vi "Release.vi"(8 "error in":errorcluster, 11 "Loop Data":T1={"VI Refnum"=refnum, "Timeout"=-1, "Code Data"=[], "Buffer Data"={"Connection ID"=refnum}, "Timer"=4294967295, "Image"=refnum}) -> (0 "error out":errorcluster)   [LabVIEW 2016]
uses:
  Data Def/Loop Data.ctl
  Com/Matrix220/Data Def/Com_Matrix220_Buffer Data.ctl
  <vilib>/vision/Image Controls.llb/IMAQ Image.ctl
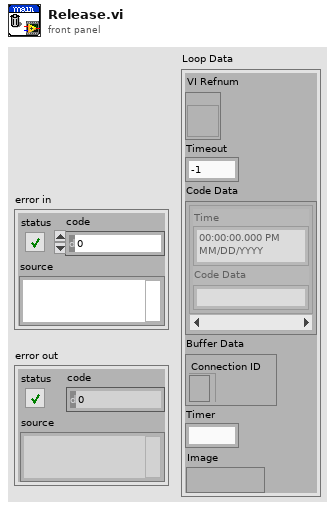
[diagram p1: front panel]
types:
  T1 = typedef "Loop Data.ctl" = cluster{"VI Refnum":refnum<vi>, "Timeout":i32, "Code Data":cluster{"Time":timestamp, "Code Data":string}[], "Buffer Data":T2, "Timer":u32, "Image":T3}
  T2 = typedef "Com_Matrix220_Buffer Data.ctl" = cluster{"Connection ID":refnum<k5>}
  T3 = typedef "IMAQ Image.ctl" = refnum<image>
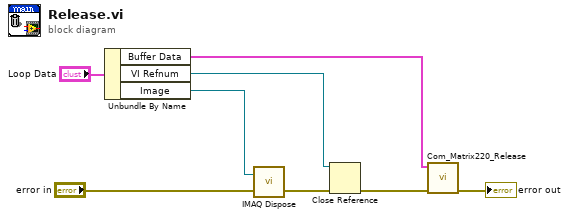
[diagram p0: block diagram]
diagram:
  n1 = Unbundle By Name("Loop Data") -> ("Buffer Data"=w5:T2, "VI Refnum"=w7:refnum<vi>, "Image"=w2:T3)
  n2 = call "IMAQ Dispose"("Image"=w2, "error in (no error)"="error in") -> ("error out"=w1:errorcluster)  [unwired: 4 in]
  n3 = Close Reference(reference=w7, error in (no error)=w1) -> (error out=w6:errorcluster)
  n4 = call "Com_Matrix220_Release.vi"("error in"=w6, "Buffer Data"=w5) -> ("error out"=→"error out":errorcluster)  [unwired: 9 in]
